vi "frequency(SubVI).vi"   [LabVIEW 2017]
uses:
  Global pulses.vi
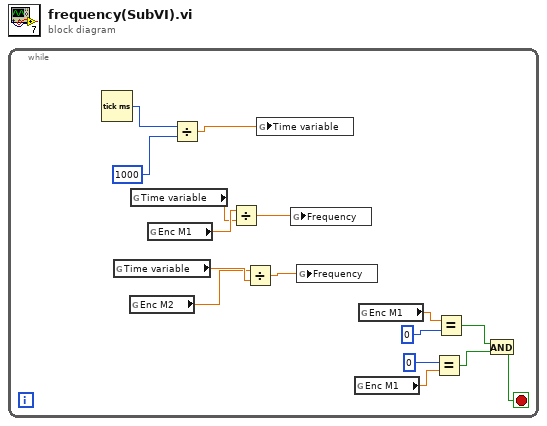
[diagram p0: block diagram]
diagram:
  n1 = while {
    stop <- w7 stop-if-true
    n2 = Tick Count (ms)() -> (millisecond timer value=w16:u32)
    n3 = global read "Global pulses.vi" "Time variable"() -> (w2:dbl)
    n4 = global read "Global pulses.vi" "Enc M2"() -> (w1:dbl)
    n5 = global read "Global pulses.vi" "Time variable"() -> (w3:dbl)
    n6 = global read "Global pulses.vi" "Enc M1"() -> (w4:dbl)
    n7 = Divide(x=w16, y=1000) -> (x/y=w14:dbl)
    n8 = Divide(x=w4, y=w3) -> (x/y=w6:dbl)
    n9 = Divide(x=w1, y=w2) -> (x/y=w5:dbl)
    n10 = global write "Global pulses.vi" "Time variable"(w14) -> ()
    n11 = global write "Global pulses.vi" "Frequency"(w6) -> ()
    n12 = global write "Global pulses.vi" "Frequency"(w5) -> ()
    n13 = global read "Global pulses.vi" "Enc M1"() -> (w10:dbl)
    n14 = global read "Global pulses.vi" "Enc M1"() -> (w11:dbl)
    n15 = Equal?(x=0, y=w10) -> (x = y?=w8:bool)
    n16 = Equal?(x=w11, y=0) -> (x = y?=w9:bool)
    n17 = And(x=w9, y=w8) -> (x .and. y?=w7:bool)
  }
